vi "State Enter Core.vi"(8 "error in":errorcluster, 11 "B State in":refnum<class "B State.lvclass">) -> (0 "error out":errorcluster, 3 "B State out":refnum<class "B State.lvclass">)   [LabVIEW 2021, in "Context.lvlib" / "B State.lvclass"]
uses:
  B State.lvclass
  B State.lvclass/B State.ctl
  Context/Context.lvclass
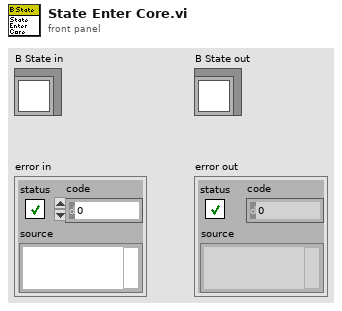
[diagram p1: front panel]
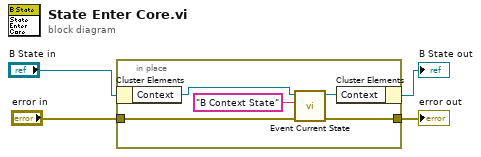
[diagram p0: block diagram]
diagram:
  n1 = in-place {
    in-place-border: "error in" -> [w7]
    in-place-border: [w6] -> w4
    n2 = in-place-cluster #1("B State in") -> ("Context"=w9:refnum<class "Context.lvclass">)
    n3 = call "Event Current State.vi"("error in"=w7, "Current State"="B Context State", "Context in"=w9) -> ("error out"=w6:errorcluster, "Context out"=w8:refnum<class "Context.lvclass">)  [unwired: 7 in]
    n4 = in-place-cluster #1("Context"=w8) -> (→"B State out":refnum<class "B State.lvclass">)
  }
  "error out" <- w4
